vi "test_raptor.vi"() -> ()   [LabVIEW 2016]
doc: "Test Raptor by pre-loading a stack of images and then sending them to Raptor, simulating an OCT acquisition system.\n\nMike Hughes, Applied Optics Group, University of Kent"
uses:
  lib/typedef/raptor_parameters.ctl
  <vilib>/Platform/TimedLoop/XDataNode/timing_clust.ctl
  <vilib>/Platform/TimedLoop/XDataNode/nitl_modes.ctl
  <vilib>/Platform/TimedLoop/XDataNode/wakeup.ctl
  <vilib>/platform/TimedLoop/XDataNode/XDataNode.xnode
  <vilib>/Platform/TimedLoop/XDataNode/XDNodeRunTimeDep.lvlib
  <vilib>/vision/NI_Vision_Development_Module.lvlib
panel:
  in  "Raptor Parameters":T1={"Vertical Search Range"=20, "Template Width"=180, "Template Height"=100, "Correlation Threshold"=0.5, "Surface Morph Size"=10, "En Face Width"=400, "En Face Height"=600, "En Face Depth"=15, "Aspect Ratio"=1.1, "Continous Scan"=FALSE, "Num En Face Reviews"=10, "Fluoresence Channel"=TRUE, "Track Depth"=TRUE, "Auto Expand"=TRUE, "Show Raptor Window"=TRUE, "Surface Threshold"=2, "Gaussian Filter Size"=1.5, "Mean Filter Size"=5.0}
  out "Lag":i64
  in  "Max Images to Load":i32=1000
  in  "TIF File for Simulated Raw Fluorescence":path
  in  "Stop Assembly":bool
  out "Current Image Sent":i64=1000
  out "Fluroescence":T2(plugin-control)
  in  "New Scan":bool
  out "B-Scan":T2(plugin-control)
  out "En Face":T2(plugin-control)
  in  "Simulated FPS":i32=250
  in  "stop":bool
  out "Num Images":i32=1000
  in  "Folder of TIFs for Simulated Raw B Scan Images":path
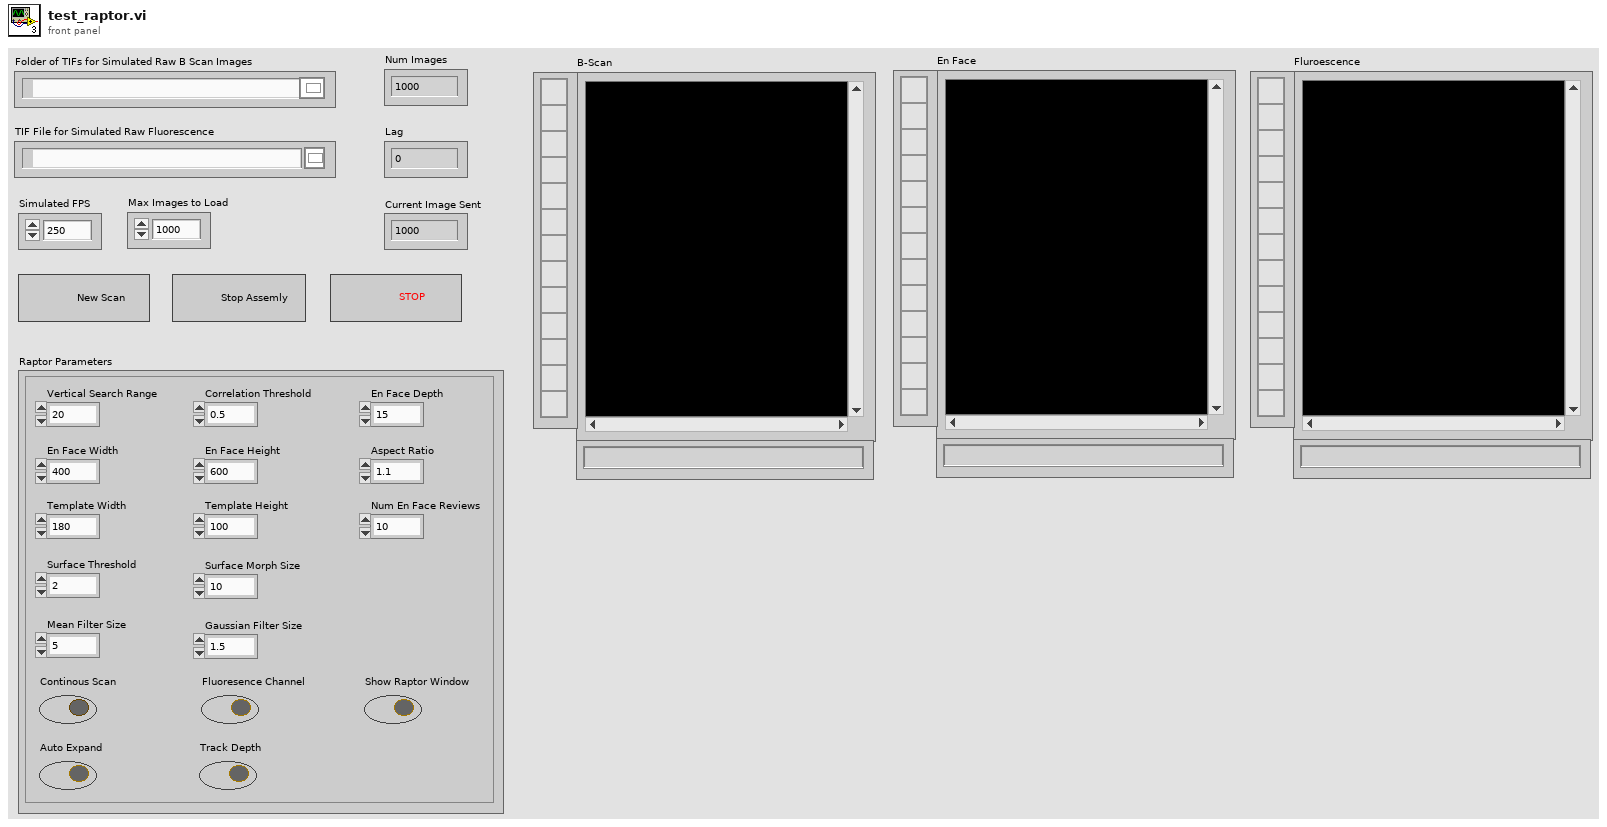
[diagram p1: front panel]
types:
  T1 = typedef "raptor_parameters.ctl" = cluster{"Vertical Search Range":i32, "Template Width":i32, "Template Height":i32, "Correlation Threshold":dbl, "Surface Morph Size":i32, "En Face Width":i32, "En Face Height":i32, "En Face Depth":i32, "Aspect Ratio":dbl, "Continous Scan":bool, "Num En Face Reviews":i32, "Fluoresence Channel":bool, "Track Depth":bool, "Auto Expand":bool, "Show Raptor Window":bool, "Surface Threshold":i32, "Gaussian Filter Size":dbl, "Mean Filter Size":dbl}
  T2 = typedef "IMAQ Image.ctl" = refnum<image>
  T3 = typedef "Image Type" = u32
  T4 = typedef "XDNodeRunTimeDep.lvlib/timing_clust.ctl" = cluster{"Expected End [f-1]":u64, "Actual End [f-1]":u64, "Finished Late? [f-1]":bool, "Expected End [i-1]":u64, "Actual End [i-1]":u64, "Finished Late? [i-1]":bool, "Expected Start [i]":u64, "Actual Start [i]":u64, "Expected Start [f]":u64, "Actual Start [f]":u64, "Source Name":string, "Structure Name":string, "Period":i64, "Deadline":i64, "Offset":i64, "Start":i64, "Priority":i32, "Timeout":i32, "Mode":T5, "Wakeup Reason":T6, "Error":errorcluster, "Source Type":string, "Secondary Source Type":string, "Global End Time":u64, "Global Start Time":u64, "Frame Duration":u64, "Iteration Duration":u64, "Assigned CPU":i32, "I/O Scan Engine Mode":u32}
  T5 = typedef "XDNodeRunTimeDep.lvlib/nitl_modes.ctl" = enum32{"No Change", "Process missed periods, maintain original phase", "Discard missed periods, maintain original phase", "Process missed periods, ignore original phase", "Discard missed periods, ignore original phase"}
  T6 = typedef "XDNodeRunTimeDep.lvlib/wakeup.ctl" = enum32{"Normal", "Aborted", "Asynchronous wakeup", "Timing source error", "Timed loop error", "Timeout"}
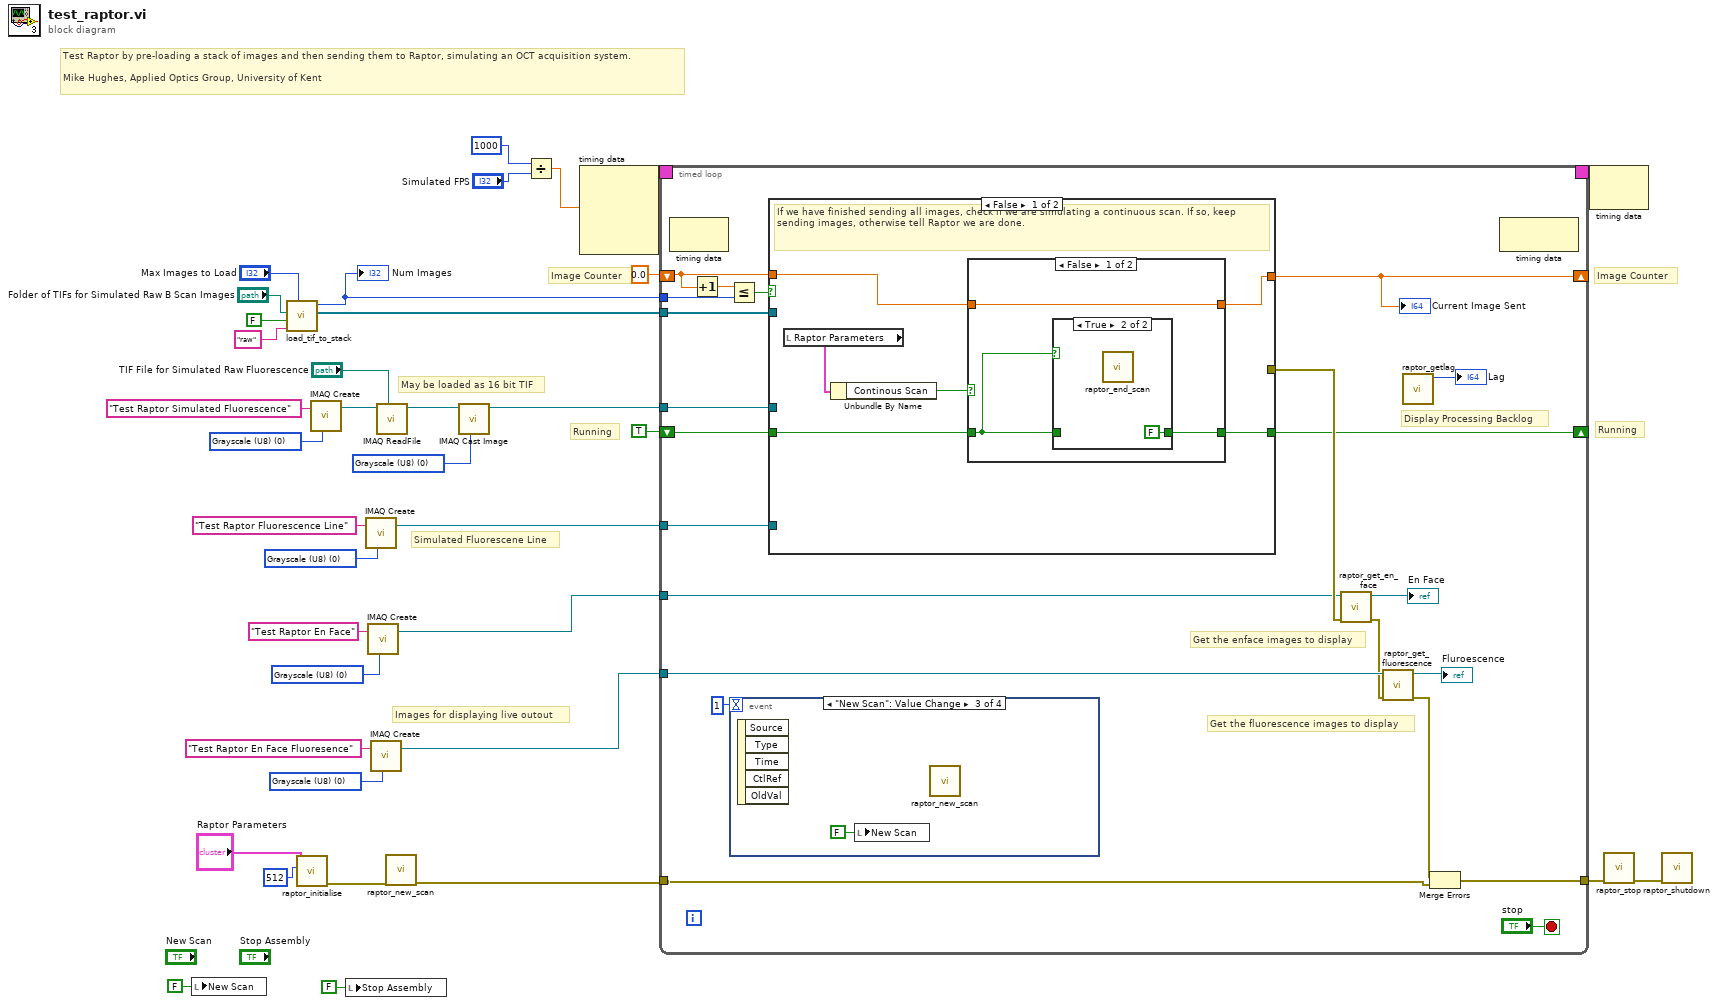
[diagram p0: block diagram]
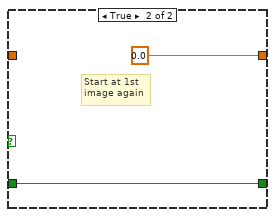
[diagram p3: hidden frame]
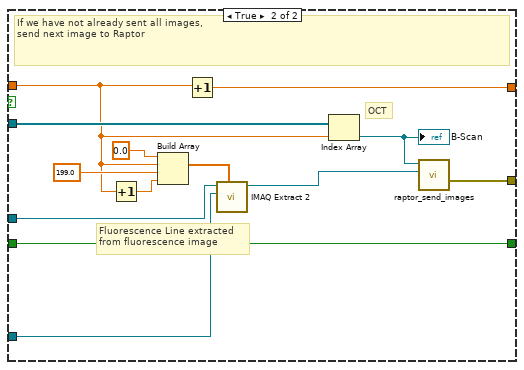
[diagram p4: hidden frame]
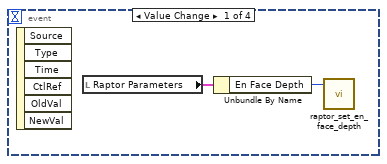
[diagram p5: hidden frame]
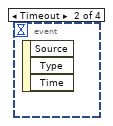
[diagram p6: hidden frame]
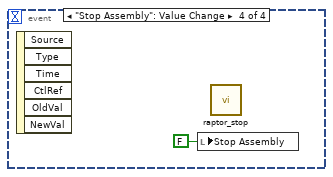
[diagram p7: hidden frame]
diagram:
  w4 = T3 0 items=["Grayscale (U8)", "Grayscale (I16)", "Grayscale (SGL)", "Complex (CSG)", "RGB (U32)", "HSL (U32)", "RGB (U64)", "Grayscale (U16)"] ("Image Type")
  w8 = T3 0 items=["Grayscale (U8)", "Grayscale (I16)", "Grayscale (SGL)", "Complex (CSG)", "RGB (U32)", "HSL (U32)", "RGB (U64)", "Grayscale (U16)"] ("Image Type")
  w19 = T3 0 items=["Grayscale (U8)", "Grayscale (I16)", "Grayscale (SGL)", "Complex (CSG)", "RGB (U32)", "HSL (U32)", "RGB (U64)", "Grayscale (U16)"] ("Image Type")
  w21 = T3 0 items=["Grayscale (U8)", "Grayscale (I16)", "Grayscale (SGL)", "Complex (CSG)", "RGB (U32)", "HSL (U32)", "RGB (U64)", "Grayscale (U16)"] ("Image Type")
  w25 = T3 0 items=["Grayscale (U8)", "Grayscale (I16)", "Grayscale (SGL)", "Complex (CSG)", "RGB (U32)", "HSL (U32)", "RGB (U64)", "Grayscale (U16)"] ("Image Type")
  # "Test Raptor by pre-loading a stack of images and then sending them to Raptor, simulating an OCT acquisition system.\n\nMike Hughes, Applied Optics Group, University of Kent"
  # "May be loaded as 16 bit TIF"
  # "Running"
  # "Simulated Fluorescene Line"
  # "Images for displaying live outout"
  # "Running"
  # "Image Counter"
  # "Image Counter"
  n1 = local write "New Scan"(FALSE ("New Scan")) -> ()
  n2 = call "load_tif_to_stack.vi"("Num Images"="Max Images to Load", "Image Prefix"="raw", "Preview"=FALSE, "TIF Files"="Folder of TIFs for Simulated Raw B Scan Images") -> ("Image Array"=w34:T2[], "Num Images"=w15:i32)  [unwired: 6 in]
  "Num Images" <- w15
  n3 = call "raptor_initialise.vi"("Buffer Size"=512, "Raptor Parameters"="Raptor Parameters") -> ("error out"=w23:errorcluster)  [unwired: 9 in]
  n4 = call "IMAQ Create"("Image Name"="Test Raptor Simulated Fluorescence", "Image Type"=w21) -> ("New Image"=w11:T2)  [unwired: 3 in, 1 out]
  n5 = local write "Stop Assembly"(FALSE ("Stop Assembly")) -> ()
  n6 = call "IMAQ Create"("Image Name"="Test Raptor Fluorescence Line", "Image Type"=w8) -> ("New Image"=w7:T2)  [unwired: 3 in, 1 out]
  n7 = call "IMAQ Create"("Image Name"="Test Raptor En Face", "Image Type"=w25) -> ("New Image"=w24:T2)  [unwired: 3 in, 1 out]
  n8 = call "IMAQ Create"("Image Name"="Test Raptor En Face Fluoresence", "Image Type"=w19) -> ("New Image"=w17:T2)  [unwired: 3 in, 1 out]
  n9 = call "IMAQ ReadFile"("File Path"="TIF File for Simulated Raw Fluorescence", "Image"=w11) -> ("Image Out"=w6:T2)  [unwired: 5 in, 4 out]
  n10 = call "raptor_new_scan.vi"("error in (no error)"=w23) -> ("error out"=w22:errorcluster)  [unwired: 10 in]
  n11 = call "IMAQ Cast Image"("Image Type"=w4, "Image Src"=w6) -> ("Image Dst Out"=w5:T2)  [unwired: 8 in, 1 out]
  n12 = Divide(x=1000, y="Simulated FPS") -> (x/y=w27:dbl)
  n13 = node-c288(w27) -> (w31:T4)  [unwired: 3 in]
  n14 = timed-loop {
    tunnel: w34 -> [w59]
    tunnel: [w50] -> w32
    tunnel: w22 -> [w52]
    timing: w31 -> [_]
    timing-out: [_] -> w30
    tunnel: w24 -> [w56]
    tunnel: w5 -> [w49]
    tunnel: w17 -> [w54]
    tunnel: w15 -> [w48]
    shift-right: [w46] -> _
    shift-left: sgl 0.0 ("Pixel Value (U8, U16, I16, Float)") -> [w42]
    shift-right: [w44] -> _
    shift-left: TRUE -> [w45]
    tunnel: w7 -> [w41]
    stop <- "stop" stop-if-true
    # "Display Processing Backlog"
    # "Get the fluorescence images to display"
    # "Get the enface images to display"
    n15 = node-c288() -> ()  [unwired: 1 in, 1 out]
    n16 = Increment(x=w42) -> (x+1=w43:sgl)
    n17 = Less Or Equal?(x=w43, y=w48) -> (x <= y?=w47:bool)
    n18 = event shown="[2] \"New Scan\": Value Change" {
      selector: _ -> [_ _ _ _]
      dyn-events: _ -> [_ _ _ _]
      timeout: 1 -> [_ _ _ _]
      event Value Change {
        n19 = event-data() -> ()  [unwired: 1 in, 6 out]
        n20 = local read "Raptor Parameters"() -> (w87:T1)
        n21 = Unbundle By Name(w87) -> ("En Face Depth"=w86:i32)
        n22 = call "raptor_set_en_face_depth.vi"("Depth"=w86) -> ()  [unwired: 10 in, 1 out]
      }
      event Timeout {
        n23 = event-data() -> ()  [unwired: 1 in, 3 out]
      }
      event "New Scan": Value Change {
        n24 = event-data() -> ()  [unwired: 1 in, 5 out]
        n25 = local write "New Scan"(FALSE ("New Scan")) -> ()
        n26 = call "raptor_new_scan.vi"() -> ()  [unwired: 11 in, 1 out]
      }
      event "Stop Assembly": Value Change {
        n27 = event-data() -> ()  [unwired: 1 in, 6 out]
        n28 = local write "Stop Assembly"(FALSE ("Stop Assembly")) -> ()
        n29 = call "raptor_stop.vi"() -> ()  [unwired: 11 in, 1 out]
      }
    }
    n30 = case shown="False" w47 {
      tunnel: w59 -> [_ w85]
      tunnel: [_ w84] -> w57
      tunnel: w49 -> [_ w80]
      tunnel: w42 -> [w65 w73]
      tunnel: [w64 w82] -> w46
      tunnel: w45 -> [w62 w81]
      tunnel: [w61 w81] -> w44
      tunnel: w41 -> [_ w79]
      frame False {
        # "If we have finished sending all images, check if we are simulating a continuous scan. If so, keep sending images, otherwise tell Raptor we are done."
        n31 = local read "Raptor Parameters"() -> (w60:T1)
        n32 = Unbundle By Name(w60) -> ("Continous Scan"=w63:bool)
        n33 = case shown="False" w63 {
          tunnel: w65 -> [w68 _]
          tunnel: [w68 sgl 0.0 ("Pixel Value (U8, U16, I16, Float)")] -> w64
          tunnel: w62 -> [w67 w71]
          tunnel: [w66 w71] -> w61
          frame False {
            n34 = case shown="True" w67 {
              tunnel: w67 -> [w69 _]
              tunnel: [w69 FALSE] -> w66
              frame False {
              }
              frame True {
                n35 = call "raptor_end_scan.vi"() -> ()  [unwired: 11 in, 1 out]
              }
            }
          }
          frame True {
            # "Start at 1st \nimage again"
          }
        }
      }
      frame True {
        # "Fluorescence Line extracted \nfrom fluorescence image"
        # "OCT"
        # "If we have not already sent all images, \nsend next image to Raptor"
        n36 = Increment(x=w73) -> (x+1=w74:sgl)
        n37 = Build Array(0.0 ("element"), w73, 199.0 ("element"), w74) -> (w78:dbl[])
        n38 = Increment(x=w73) -> (x+1=w82:sgl)
        n39 = call "IMAQ Extract 2"("Optional Rectangle"=w78, "Image Dst"=w79, "Image Src"=w80) -> ("Image Dst Out"=w75:T2)  [unwired: 7 in, 1 out]
        n40 = Index Array(array=w85, index=w73) -> (element=w83:T2)
        "B-Scan" <- w83
        n41 = call "raptor_send_images.vi"("Image Channel 2"=w75, "Image Channel 1"=w83) -> ("error out"=w84:errorcluster)  [unwired: 9 in]
      }
    }
    "Current Image Sent" <- w46
    n42 = call "raptor_get_en_face.vi"("error in (no error)"=w57, "Image Src"=w56) -> ("error out"=w53:errorcluster, "Image Dst Out"=→"En Face":T2)  [unwired: 8 in]
    n43 = call "raptor_get_fluorescence.vi"("error in (no error)"=w53, "Image Src"=w54) -> ("error out"=w51:errorcluster, "Image Dst Out"=→"Fluroescence":T2)  [unwired: 8 in]
    n44 = call "raptor_getlag.vi"() -> ("Frame Lag"=→"Lag":i32)  [unwired: 10 in, 1 out]
    n45 = Merge Errors(w51, w52) -> (w50:errorcluster)
    n46 = node-c288() -> ()  [unwired: 1 in, 1 out]
  }
  n47 = node-c288(w30) -> ()  [unwired: 1 out]
  n48 = call "raptor_stop.vi"("error in (no error)"=w32) -> ("error out"=w33:errorcluster)  [unwired: 10 in]
  n49 = call "raptor_shutdown.vi"("error in (no error)"=w33) -> ()  [unwired: 10 in, 1 out]
